vi "VNA_Interferometer.vi"() -> ()   [LabVIEW 2015]
doc: "Measure VNA FMR with interferometer circuit."
uses:
  <vilib>/Utility/file.llb/Read Delimited Spreadsheet (DBL).vi
  <vilib>/Utility/file.llb/Write Delimited Spreadsheet (DBL).vi
  <vilib>/Utility/file.llb/Write Delimited Spreadsheet (string).vi
panel:
  in  "Find fitting freq":bool
  in  "Fitting Freq":dbl=0.04650776797841169
  in  "Stopping":bool
  out "Field values":dbl[](array[numeric])
  out "Im values":dbl[](array[numeric])
  out "Re values":dbl[](array[numeric])
  in  "Polynomial Coefficients":dbl[](array[numeric])
  out "Max Field":dbl
  out "Time Remaining (min)":dbl
  out "Elapsed Time (min)":dbl caption="Elapsed Time (s)"
  in  "Trigger Delay (ms)":dbl=50.0
  in  "Burst Count":dbl=205.0
  in  "Modulation Frequency (Hz)":dbl=47.0
  in  "Amplitide (V)":dbl=5.0
  in  "SG GPIB Address":i16=22
  out "Total Points":dbl
  out "Field Set (Oe)":dbl
  in  "Start":bool
  out "Ready":bool
  in  "Stop":bool
  out "Status":string
  out "Measurement #":dbl
  out "Field Read (Oe)":dbl
  out "Email Errors":string
  out "Im Measurements":cluster{dbl[], dbl[]}(graph)
  out "Re Measurements":cluster{dbl[], dbl[]}(graph)
  out "Im VNA Output":cluster{"X-values":dbl[], "Input data":dbl[]}[](graph)
  in  "VNA Points":dbl=1000.0
  in  "VNA Power (dBm)":string="-17"
  in  "VNA GPIB Address":refnum<visa-resource-name>="GPIB0::15::INSTR"
  in  "VNA Frequency (GHz)":dbl=10.0
  in  "IF Bandwidth (Hz)":dbl=1000.0
  out "Re VNA Output":cluster{"X-values":dbl[], "Input data":dbl[]}[](graph)
  in  "Email Address":string
  in  "Send Email?":bool
  in  "File Name Comment":string
  in  "Save Directory":path=path "C:/Users/probe_station/Desktop/VNA_Interferometer_Data"
  in  "Gaussmeter GPIB Address":string="12"
  in  "Calibrate PS":bool
  in  "Stabilization Time (s)":dbl=5.0
  in  "Field Step (Oe)":dbl=10.0
  in  "Field Sweep Stop (Oe)":dbl=2000.0
  in  "Field Sweep Start (Oe)":dbl=5000.0
  in  "PS GPIB Address":string="1"
  # "Output Indicators"
  # "Timers"
  # "Signal Generator Controls"
  # "Program controls and status"
  # "VNA Controls"
  # "Output Controls"
  # "Field and Power Supply Controls"
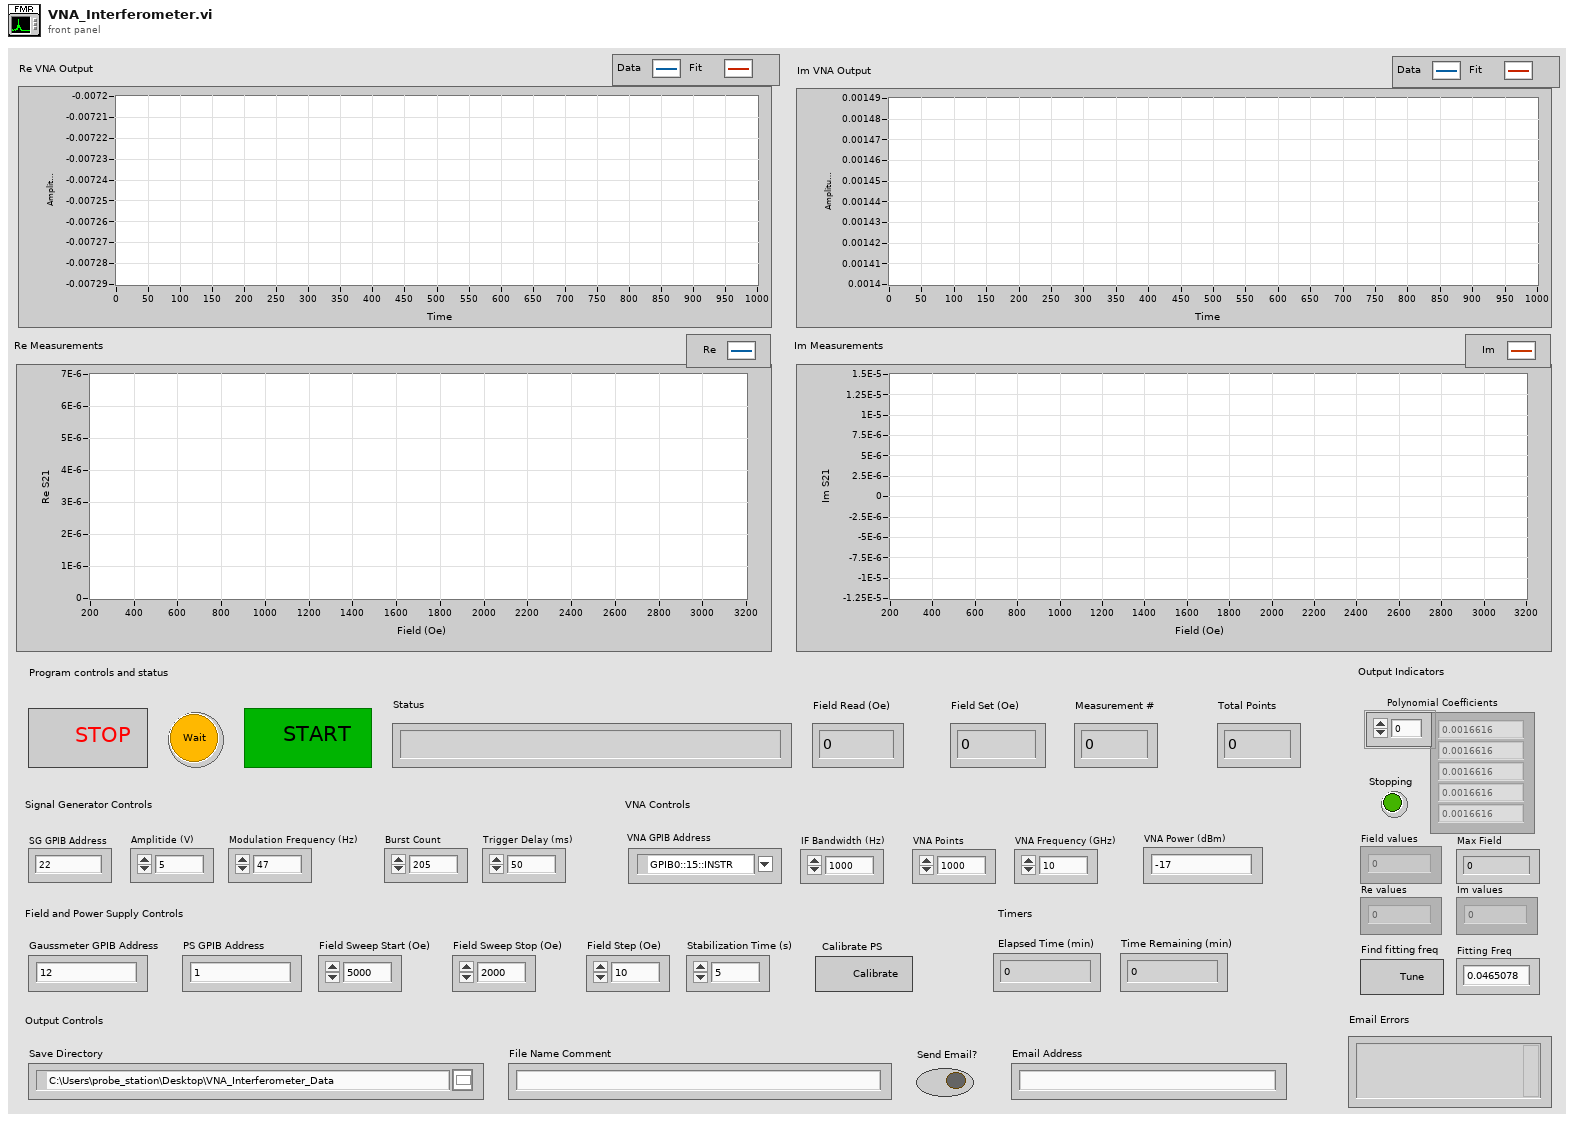
[diagram p1: front panel]
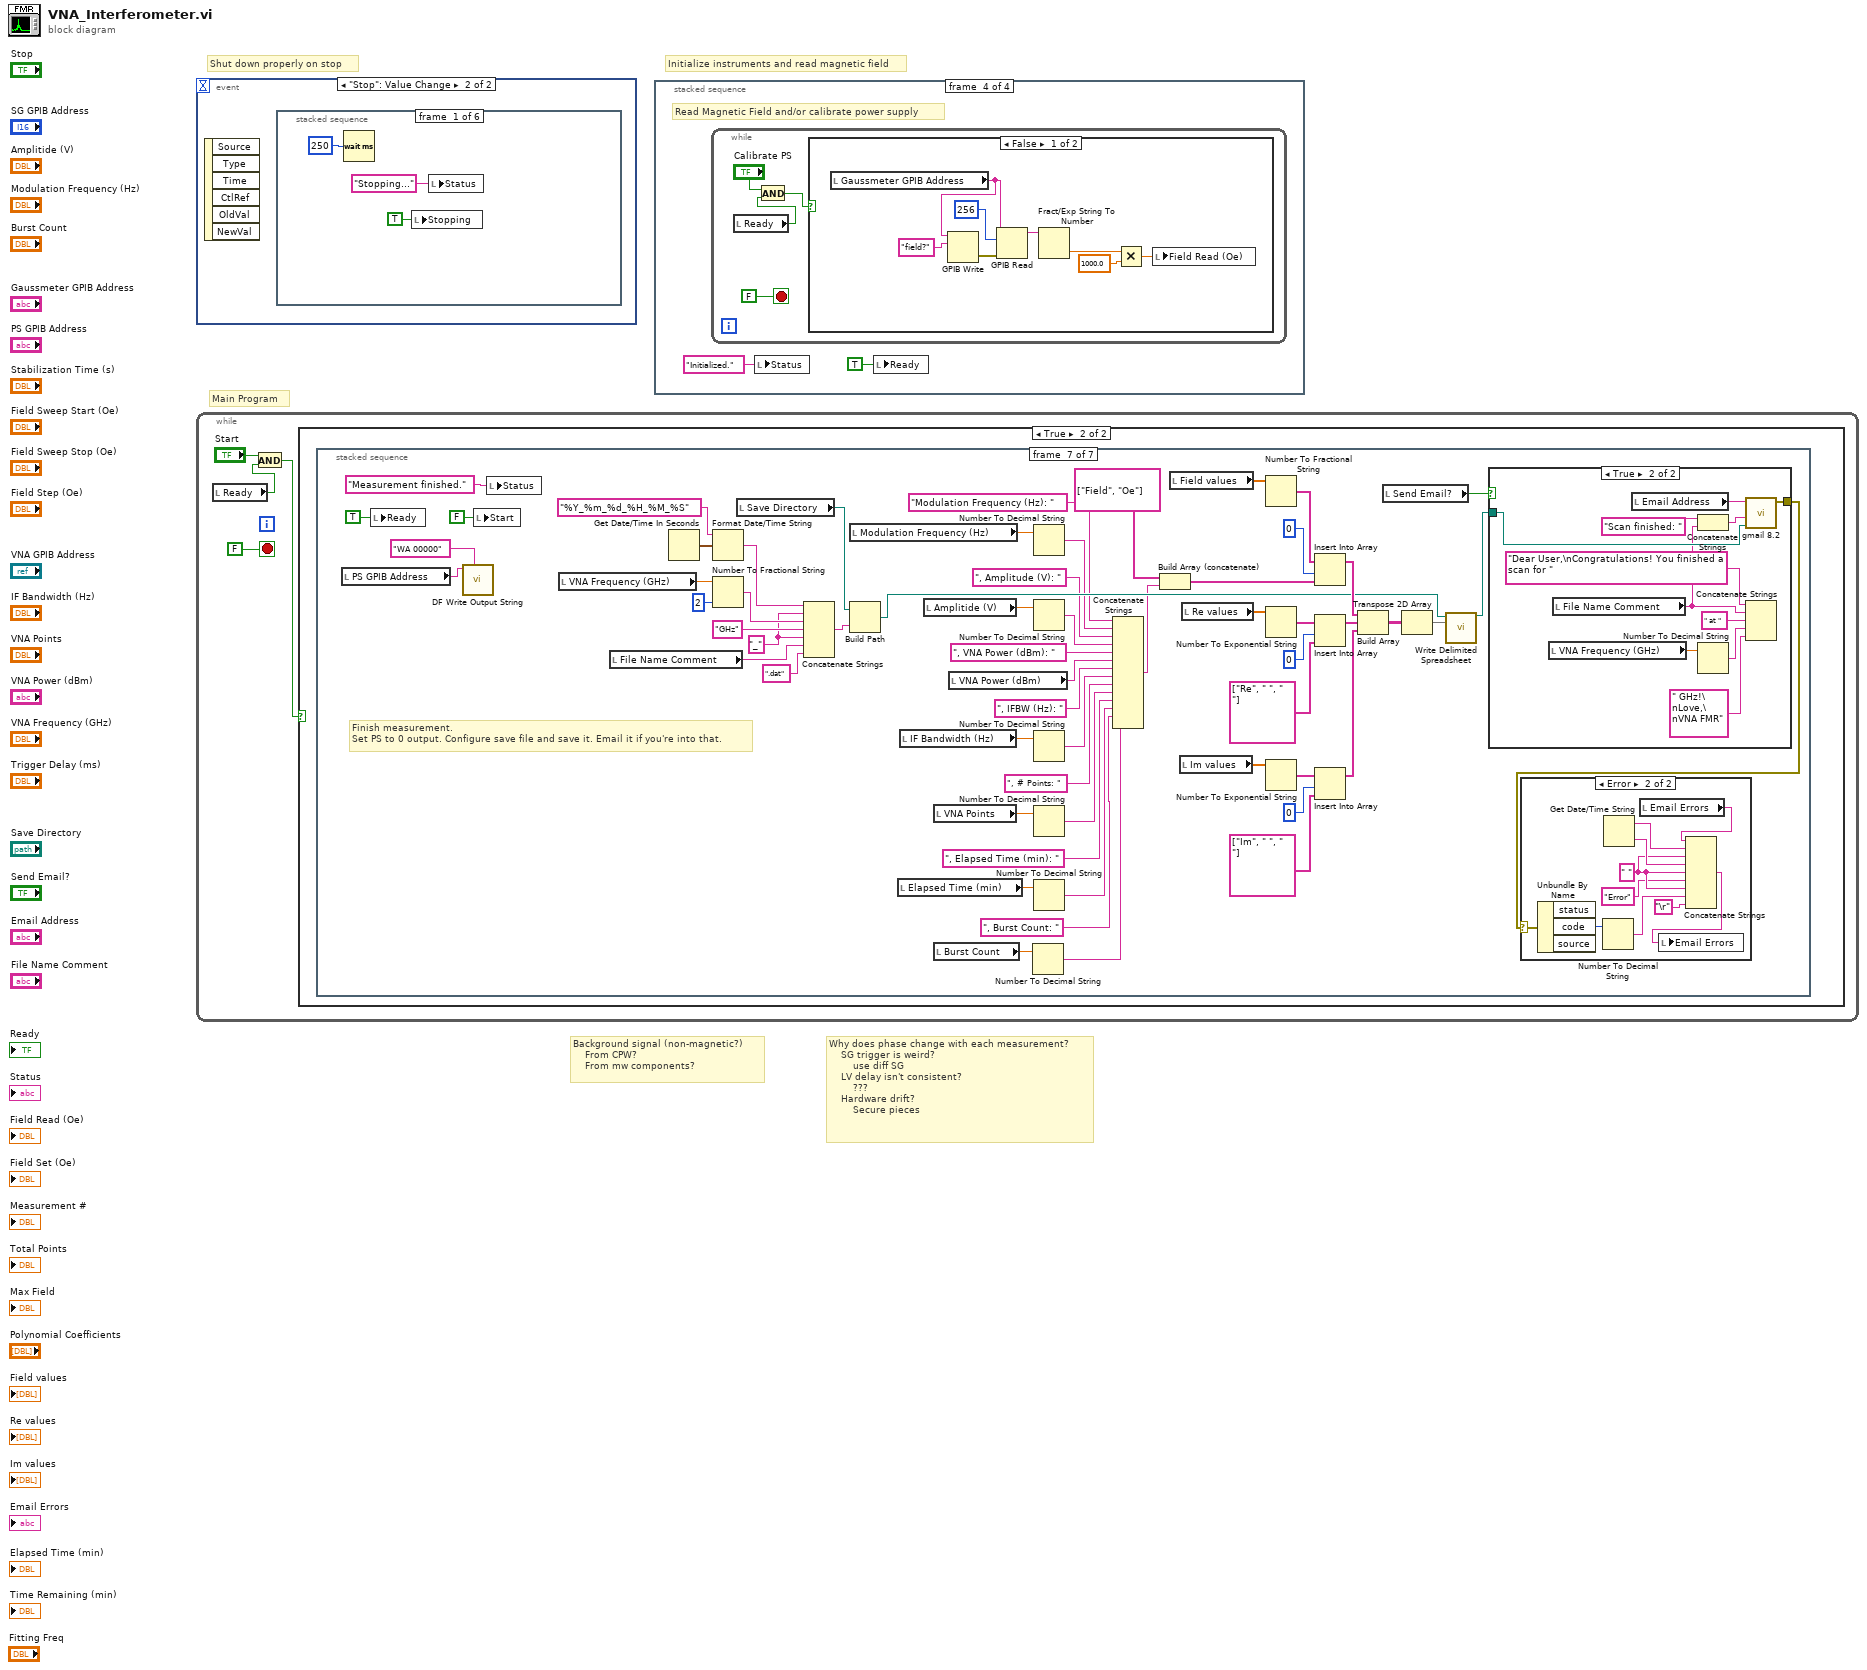
[diagram p0: block diagram]
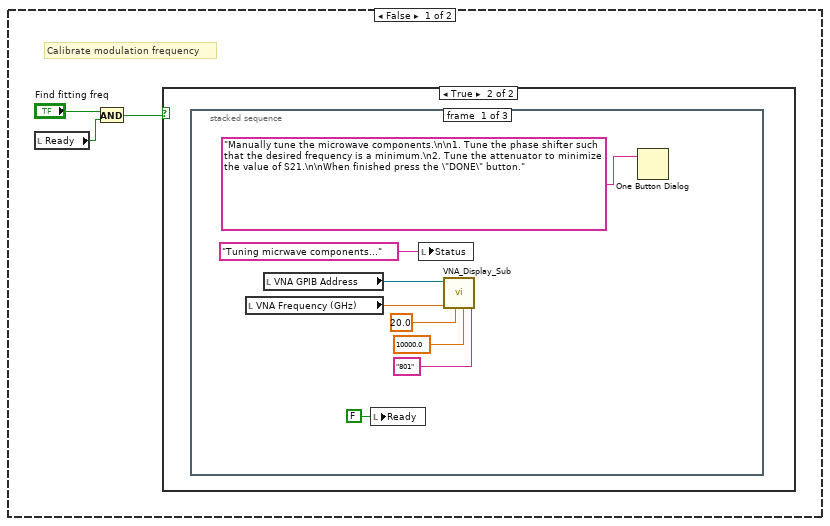
[diagram p2: hidden frame]
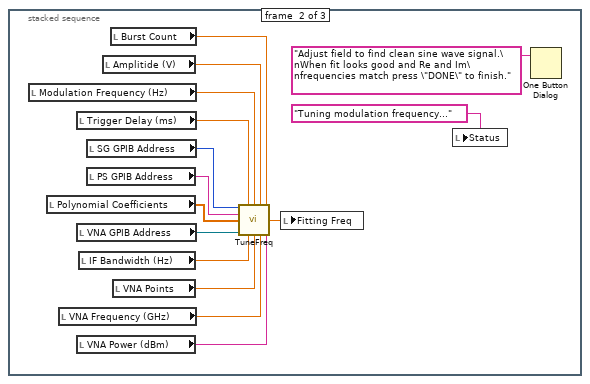
[diagram p4: hidden frame]
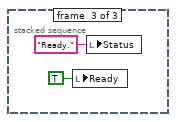
[diagram p5: hidden frame]
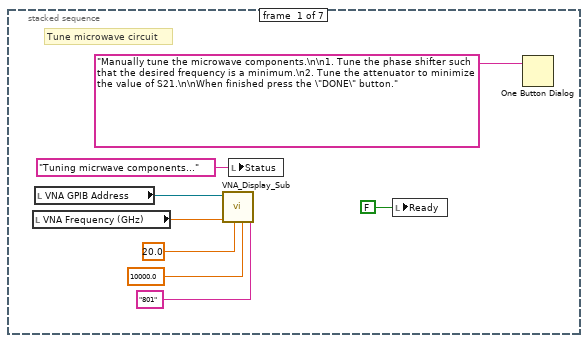
[diagram p6: hidden frame]
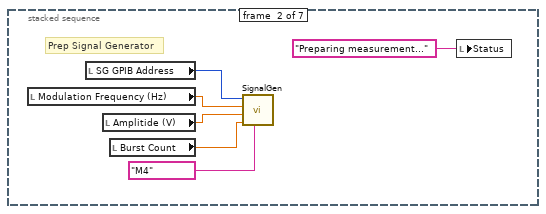
[diagram p7: hidden frame]
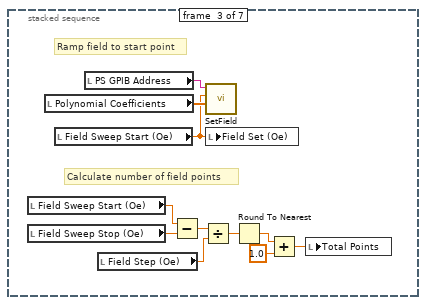
[diagram p8: hidden frame]
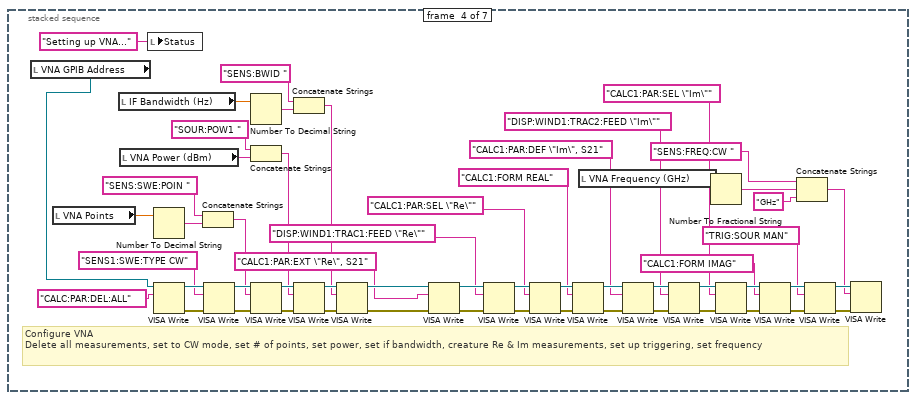
[diagram p9: hidden frame]
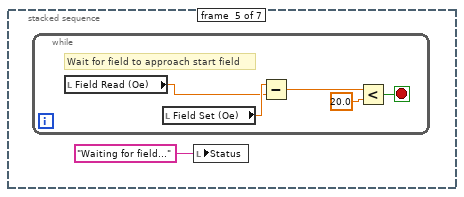
[diagram p10: hidden frame]
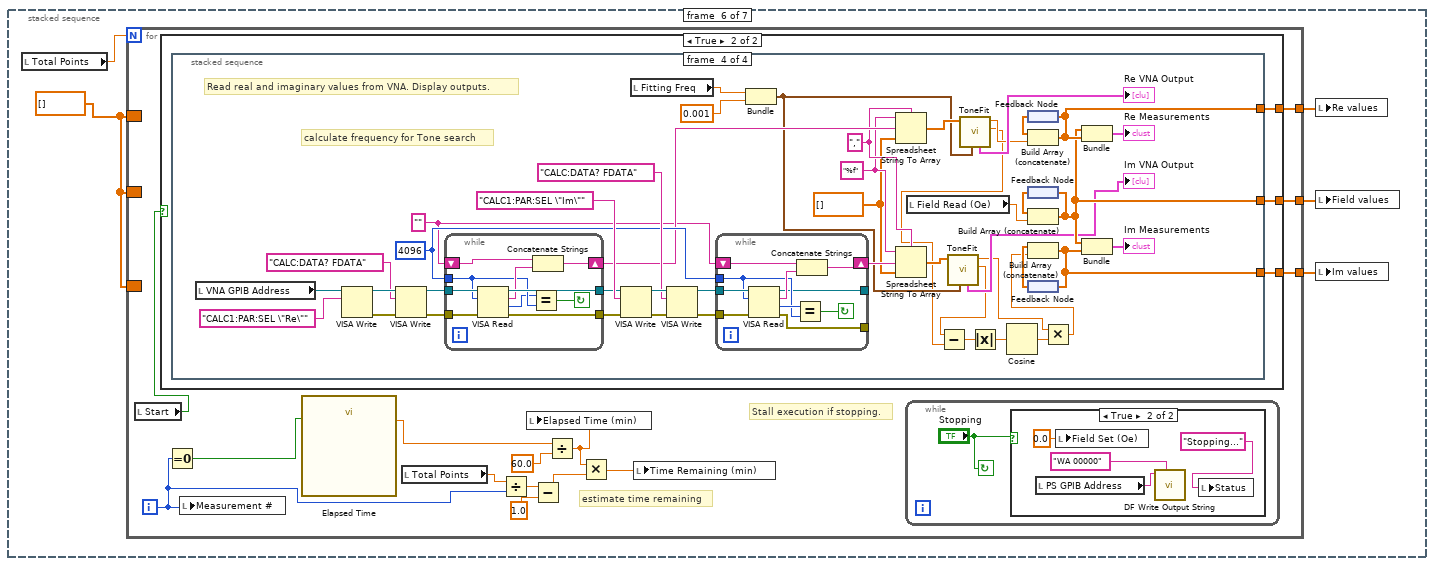
[diagram p11: hidden frame]
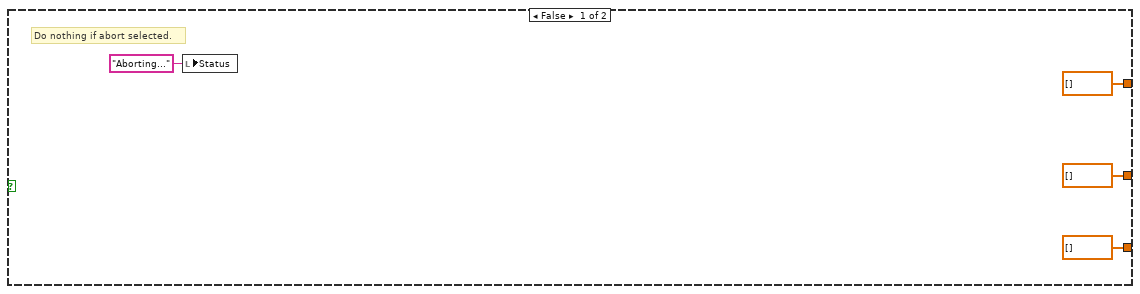
[diagram p12: hidden frame]
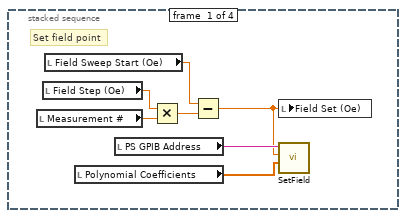
[diagram p13: hidden frame]
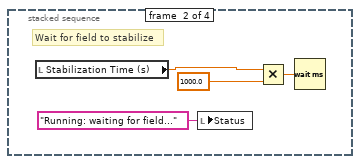
[diagram p14: hidden frame]
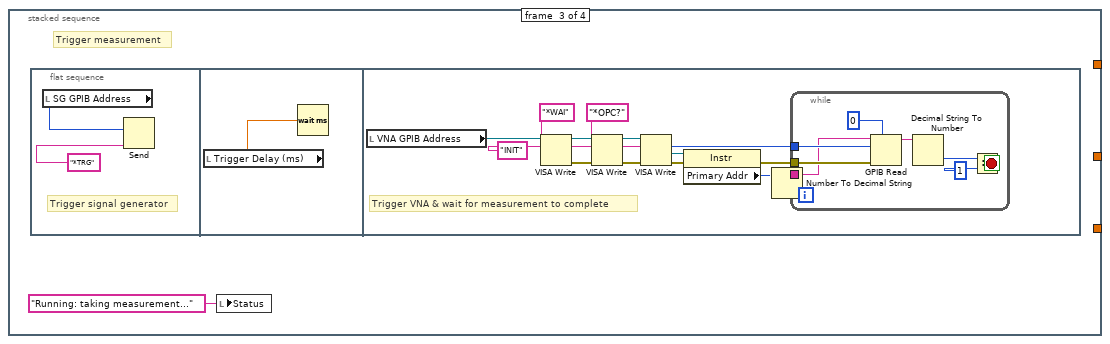
[diagram p15: hidden frame]
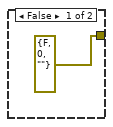
[diagram p18: hidden frame]
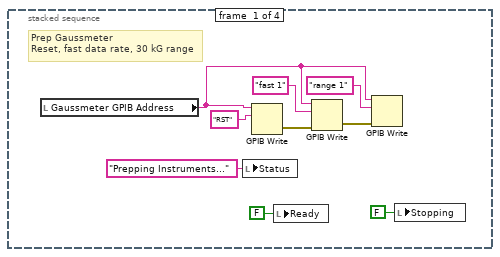
[diagram p19: hidden frame]
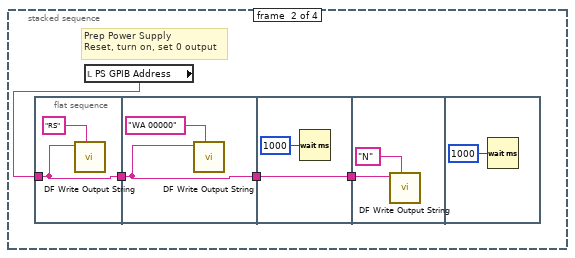
[diagram p20: hidden frame]
diagram:
  # "Background signal (non-magnetic?)\n    From CPW?\n    From mw components?"
  # "Why does phase change with each measurement?\n    SG trigger is weird?\n        use diff SG\n    LV delay isn't consistent?\n        ???\n    Hardware drift?\n        Secure pieces"
  # "Main Program"
  # "Initialize instruments and read magnetic field"
  # "Shut down properly on stop"
  n1 = event shown="[1] \"Stop\": Value Change" {
    selector: _ -> [_ _]
    dyn-events: _ -> [_ _]
    timeout: _ -> [_ _]
    event Timeout {
      n2 = event-data() -> ()  [unwired: 1 in, 3 out]
    }
    event "Stop": Value Change {
      n3 = event-data() -> ()  [unwired: 1 in, 6 out]
      n4 = stacked-sequence {
        frame #0 {
          n5 = Wait (ms)(milliseconds to wait=u32 250) -> ()  [unwired: 1 out]
          n6 = local write "Stopping"(TRUE ("Stopping")) -> ()
          n7 = local write "Status"("Stopping..." ("Status")) -> ()
        }
        frame #1 {
          # "Disable SG output"
          # "set power supply to 0 output"
          n8 = local read "PS GPIB Address"() -> (w7:string)
          n9 = local read "SG GPIB Address"() -> (w6:i16)
          n10 = call "DF Write Output String"("Write String"="WA 00000", "Communications Mode"=TRUE, "Communications On/Off"=TRUE, "GPIB Address"=w7) -> ()  [unwired: 5 in]
          n11 = Send(2:w6, 5:"D1" ("data string")) -> ()  [unwired: 3 in, 3 out]
          n12 = local write "Field Set (Oe)"(0.0 ("Field Set (Oe)")) -> ()
        }
        frame #2 {
          n13 = Wait (ms)(milliseconds to wait=u32 100) -> ()  [unwired: 1 out]
        }
        frame #3 {
          # "Wait for\nfield \nto reach\nzero"
          n14 = while {
            stop <- w12 stop-if-true
            n15 = local read "Field Read (Oe)"() -> (w14:dbl)
            n16 = Less?(x=w14, y=200.0) -> (x < y?=w12:bool)
          }
        }
        frame #4 {
          # "Turn off power supply"
          n17 = local read "PS GPIB Address"() -> (w15:string)
          n18 = local write "Status"("Stopped." ("Status")) -> ()
          n19 = call "DF Write Output String"("Write String"="F", "Communications Mode"=TRUE, "Communications On/Off"=TRUE, "GPIB Address"=w15) -> ()  [unwired: 5 in]
        }
        frame #5 {
          # "end program"
          n20 = Stop(stop? (T)=TRUE) -> ()
        }
      }
    }
  }
  n21 = while {
    stop <- FALSE stop-if-true
    n22 = local read "Ready"() -> (w23:bool)
    n23 = And(x="Start", y=w23) -> (x .and. y?=w22:bool)
    n24 = case shown="True" w22 {
      frame False {
        # "Calibrate modulation frequency"
        n25 = local read "Ready"() -> (w27:bool)
        n26 = And(x="Find fitting freq", y=w27) -> (x .and. y?=w25:bool)
        n27 = case shown="True" w25 {
          frame False {
          }
          frame True {
            n28 = stacked-sequence {
              frame #0 {
                n29 = local read "VNA Frequency (GHz)"() -> (w32:dbl)
                n30 = local read "VNA GPIB Address"() -> (w33:refnum<visa-resource-name>)
                n31 = local write "Ready"(FALSE ("Ready")) -> ()
                n32 = local write "Status"("Tuning micrwave components..." ("Status")) -> ()
                n33 = call "VNA_Display_Sub.vi"("Num points"="801", "IF Bandwidth"=10000.0, "Span Frequency (MHz)"=20.0, "Center Frequency (GHz)"=w32, "VNA Address"=w33) -> ()  [unwired: 7 in]
                n34 = One Button Dialog(message="Manually tune the microwave components.\n\n1. Tune the phase shifter such that the desired frequency is a minimum.\n2. Tune the attenuator to minimize the value of S21.\n\nWhen finished press the \"DONE\" button.") -> ()  [unwired: 1 in, 1 out]
              }
              frame #1 {
                n35 = local read "Modulation Frequency (Hz)"() -> (w41:dbl)
                n36 = local read "Polynomial Coefficients"() -> (w48:dbl[])
                n37 = local read "VNA Frequency (GHz)"() -> (w44:dbl)
                n38 = local read "Trigger Delay (ms)"() -> (w42:dbl)
                n39 = local read "VNA GPIB Address"() -> (w47:refnum<visa-resource-name>)
                n40 = local read "VNA Power (dBm)"() -> (w43:string)
                n41 = local read "IF Bandwidth (Hz)"() -> (w46:dbl)
                n42 = local read "SG GPIB Address"() -> (w50:i16)
                n43 = local read "PS GPIB Address"() -> (w49:string)
                n44 = local read "Amplitide (V)"() -> (w40:dbl)
                n45 = local read "Burst Count"() -> (w39:dbl)
                n46 = local read "VNA Points"() -> (w45:dbl)
                n47 = call "TuneFreq.vi"("SG GPIB Address"=w50, "Trigger Delay"=w42, "Mod Freq (Hz)"=w41, "Amplitude (V)"=w40, "Burst count"=w39, "PS GPIB Address"=w49, "Poly Coeffs"=w48, "VNA GPIB Address"=w47, "IF Bandwidth"=w46, "VNA Points"=w45, "VNA Frequency"=w44, "VNA Power (dBm)"=w43) -> ("Re Freq"=w38:dbl)  [unwired: 3 in]
                n48 = local write "Fitting Freq"(w38) -> ()
                n49 = local write "Status"("Tuning modulation frequency..." ("Status")) -> ()
                n50 = One Button Dialog(message="Adjust field to find clean sine wave signal.\nWhen fit looks good and Re and Im\nfrequencies match press \"DONE\" to finish.") -> ()  [unwired: 1 in, 1 out]
              }
              frame #2 {
                n51 = local write "Ready"(TRUE ("Ready")) -> ()
                n52 = local write "Status"("Ready." ("Status")) -> ()
              }
            }
          }
        }
      }
      frame True {
        n53 = stacked-sequence {
          frame #0 {
            # "Tune microwave circuit"
            n54 = local read "VNA Frequency (GHz)"() -> (w58:dbl)
            n55 = local read "VNA GPIB Address"() -> (w59:refnum<visa-resource-name>)
            n56 = call "VNA_Display_Sub.vi"("Num points"="801", "IF Bandwidth"=10000.0, "Span Frequency (MHz)"=20.0, "Center Frequency (GHz)"=w58, "VNA Address"=w59) -> ()  [unwired: 7 in]
            n57 = local write "Status"("Tuning micrwave components..." ("Status")) -> ()
            n58 = local write "Ready"(FALSE ("Ready")) -> ()
            n59 = One Button Dialog(message="Manually tune the microwave components.\n\n1. Tune the phase shifter such that the desired frequency is a minimum.\n2. Tune the attenuator to minimize the value of S21.\n\nWhen finished press the \"DONE\" button.") -> ()  [unwired: 1 in, 1 out]
          }
          frame #1 {
            # "Prep Signal Generator"
            n60 = local read "Modulation Frequency (Hz)"() -> (w65:dbl)
            n61 = local read "SG GPIB Address"() -> (w66:i16)
            n62 = local read "Amplitide (V)"() -> (w64:dbl)
            n63 = local read "Burst Count"() -> (w61:dbl)
            n64 = call "SignalGen.vi"("Trigger Mode (Cont)"="M4" ("Trigger Mode"), "Burst Count"=w61, "Amplitide (V)"=w64, "Modulation Frequency (Hz)"=w65, "SG GPIB Address"=w66) -> ()  [unwired: 7 in]
            n65 = local write "Status"("Preparing measurement..." ("Status")) -> ()
          }
          frame #2 {
            # "Calculate number of field points"
            # "Ramp field to start point"
            n66 = local read "Field Sweep Start (Oe)"() -> (w72:dbl)
            n67 = local read "Field Sweep Stop (Oe)"() -> (w71:dbl)
            n68 = local read "Polynomial Coefficients"() -> (w76:dbl[])
            n69 = local read "Field Sweep Start (Oe)"() -> (w75:dbl)
            n70 = local read "PS GPIB Address"() -> (w77:string)
            n71 = local read "Field Step (Oe)"() -> (w73:dbl)
            n72 = Subtract(x=w72, y=w71) -> (x-y=w74:dbl)
            n73 = Divide(x=w74, y=w73) -> (x/y=w70:dbl)
            n74 = call "SetField.vi"("Poly Coeffs"=w76, "Field Setpoint"=w75, "PS GPIB Address"=w77) -> ()  [unwired: 9 in]
            n75 = local write "Field Set (Oe)"(w75) -> ()
            n76 = Round To Nearest(number=w70) -> (nearest integer value=w69:dbl)
            n77 = Add(x=w69, y=1.0) -> (x+y=w67:dbl)
            n78 = local write "Total Points"(w67) -> ()
          }
          frame #3 {
            # "Configure VNA\nDelete all measurements, set to CW mode, set # of points, set power, set if bandwidth, creature Re & Im measurements, set up triggering, set frequency"
            n79 = local read "VNA GPIB Address"() -> (w86:refnum<visa-resource-name>)
            n80 = local read "VNA Points"() -> (w128:dbl)
            n81 = local read "IF Bandwidth (Hz)"() -> (w117:dbl)
            n82 = local read "VNA Power (dBm)"() -> (w122:string)
            n83 = local write "Status"("Setting up VNA..." ("Status")) -> ()
            n84 = Number To Decimal String(number=w128) -> (decimal integer string=w127:string)  [unwired: 1 in]
            n85 = VISA Write(VISA resource name=w86, write buffer="CALC:PAR:DEL:ALL" ("Characters to Write")) -> (VISA resource name out=w133:refnum<visa-resource-name>, error out=w87:errorcluster)  [unwired: 1 in, 1 out]
            n86 = Concatenate Strings("SENS:SWE:POIN " ("Characters to Write"), w127) -> (w126:string)
            n87 = VISA Write(VISA resource name=w133, write buffer="SENS1:SWE:TYPE CW" ("Characters to Write"), error in (no error)=w87) -> (VISA resource name out=w130:refnum<visa-resource-name>, error out=w131:errorcluster)  [unwired: 1 out]
            n88 = Number To Decimal String(number=w117) -> (decimal integer string=w116:string)  [unwired: 1 in]
            n89 = Concatenate Strings("SOUR:POW1 " ("Characters to Write"), w122) -> (w121:string)
            n90 = VISA Write(VISA resource name=w130, write buffer=w126, error in (no error)=w131) -> (VISA resource name out=w124:refnum<visa-resource-name>, error out=w125:errorcluster)  [unwired: 1 out]
            n91 = Concatenate Strings("SENS:BWID " ("Characters to Write"), w116) -> (w115:string)
            n92 = VISA Write(VISA resource name=w124, write buffer=w121, error in (no error)=w125) -> (VISA resource name out=w119:refnum<visa-resource-name>, error out=w120:errorcluster)  [unwired: 1 out]
            n93 = VISA Write(VISA resource name=w119, write buffer=w115, error in (no error)=w120) -> (VISA resource name out=w113:refnum<visa-resource-name>, error out=w114:errorcluster)  [unwired: 1 out]
            n94 = VISA Write(VISA resource name=w113, write buffer="CALC1:PAR:EXT \"Re\", S21" ("Characters to Write"), error in (no error)=w114) -> (VISA resource name out=w110:refnum<visa-resource-name>, error out=w111:errorcluster)  [unwired: 1 out]
            n95 = VISA Write(VISA resource name=w110, write buffer="DISP:WIND1:TRAC1:FEED \"Re\"" ("Characters to Write"), error in (no error)=w111) -> (VISA resource name out=w107:refnum<visa-resource-name>, error out=w108:errorcluster)  [unwired: 1 out]
            n96 = VISA Write(VISA resource name=w107, write buffer="CALC1:PAR:SEL \"Re\"" ("Characters to Write"), error in (no error)=w108) -> (VISA resource name out=w104:refnum<visa-resource-name>, error out=w105:errorcluster)  [unwired: 1 out]
            n97 = VISA Write(VISA resource name=w104, write buffer="CALC1:FORM REAL" ("Characters to Write"), error in (no error)=w105) -> (VISA resource name out=w101:refnum<visa-resource-name>, error out=w102:errorcluster)  [unwired: 1 out]
            n98 = local read "VNA Frequency (GHz)"() -> (w80:dbl)
            n99 = VISA Write(VISA resource name=w101, write buffer="CALC1:PAR:DEF \"Im\", S21" ("Characters to Write"), error in (no error)=w102) -> (VISA resource name out=w99:refnum<visa-resource-name>, error out=w98:errorcluster)  [unwired: 1 out]
            n100 = VISA Write(VISA resource name=w99, write buffer="DISP:WIND1:TRAC2:FEED \"Im\"" ("Characters to Write"), error in (no error)=w98) -> (VISA resource name out=w95:refnum<visa-resource-name>, error out=w96:errorcluster)  [unwired: 1 out]
            n101 = Number To Fractional String(number=w80) -> (F-format string=w81:string)  [unwired: 3 in]
            n102 = VISA Write(VISA resource name=w95, write buffer="CALC1:PAR:SEL \"Im\"" ("Characters to Write"), error in (no error)=w96) -> (VISA resource name out=w92:refnum<visa-resource-name>, error out=w93:errorcluster)  [unwired: 1 out]
            n103 = VISA Write(VISA resource name=w92, write buffer="CALC1:FORM IMAG" ("Characters to Write"), error in (no error)=w93) -> (VISA resource name out=w89:refnum<visa-resource-name>, error out=w90:errorcluster)  [unwired: 1 out]
            n104 = Concatenate Strings("SENS:FREQ:CW " ("Characters to Write"), w81, "GHz" ("string")) -> (w78:string)
            n105 = VISA Write(VISA resource name=w89, write buffer="TRIG:SOUR MAN", error in (no error)=w90) -> (VISA resource name out=w83:refnum<visa-resource-name>, error out=w84:errorcluster)  [unwired: 1 out]
            n106 = VISA Write(VISA resource name=w83, write buffer=w78, error in (no error)=w84) -> ()  [unwired: 3 out]
          }
          frame #4 {
            n107 = while {
              stop <- w139 stop-if-true
              # "Wait for field to approach start field"
              n108 = local read "Field Read (Oe)"() -> (w136:dbl)
              n109 = local read "Field Set (Oe)"() -> (w137:dbl)
              n110 = Subtract(x=w137, y=w136) -> (x-y=w138:dbl)
              n111 = Less?(x=w138, y=20.0) -> (x < y?=w139:bool)
            }
            n112 = local write "Status"("Waiting for field..." ("Status")) -> ()
          }
          frame #5 {
            w144 = dbl[] []
            n113 = local read "Total Points"() -> (w145:dbl)
            n114 = for {
              N: w145 -> [_]
              border: w144 -> [_]
              border: w144 -> [_]
              border: w144 -> [_]
              tunnel: [w159] -> w143
              tunnel: [w158] -> w142
              tunnel: [w157] -> w141
              i -> [w154]
              # "estimate time remaining"
              # "Stall execution if stopping."
              n115 = local read "Start"() -> (w156:bool)
              n116 = case shown="True" w156 {
                tunnel: [dbl[] [] w166] -> w159
                tunnel: [dbl[] [] w165] -> w158
                tunnel: [dbl[] [] w164] -> w157
                frame False {
                  # "Do nothing if abort selected."
                  n117 = local write "Status"("Aborting..." ("Status")) -> ()
                }
                frame True {
                  n118 = stacked-sequence {
                    tunnel: [_ _ _ w222] -> w166
                    tunnel: [_ _ _ w221] -> w165
                    tunnel: [_ _ _ w220] -> w164
                    frame #0 {
                      # "Set field point"
                      n119 = local read "Measurement #"() -> (w169:dbl)
                      n120 = local read "Field Step (Oe)"() -> (w168:dbl)
                      n121 = local read "Field Sweep Start (Oe)"() -> (w171:dbl)
                      n122 = local read "Polynomial Coefficients"() -> (w172:dbl[])
                      n123 = local read "PS GPIB Address"() -> (w173:string)
                      n124 = Multiply(x=w168, y=w169) -> (x*y=w170:dbl)
                      n125 = Subtract(x=w171, y=w170) -> (x-y=w167:dbl)
                      n126 = local write "Field Set (Oe)"(w167) -> ()
                      n127 = call "SetField.vi"("Poly Coeffs"=w172, "Field Setpoint"=w167, "PS GPIB Address"=w173) -> ()  [unwired: 9 in]
                    }
                    frame #1 {
                      # "Wait for field to stabilize"
                      n128 = local read "Stabilization Time (s)"() -> (w176:dbl)
                      n129 = local write "Status"("Running: waiting for field..." ("Status")) -> ()
                      n130 = Multiply(x=w176, y=1000.0) -> (x*y=w175:dbl)
                      n131 = Wait (ms)(milliseconds to wait=w175) -> ()  [unwired: 1 out]
                    }
                    frame #2 {
                      # "Trigger measurement"
                      n132 = flat-sequence {
                        frame #0 {
                          # "Trigger signal generator"
                          n133 = local read "SG GPIB Address"() -> (w180:i16)
                          n134 = Send(2:w180, 5:"*TRG") -> ()  [unwired: 3 in, 3 out]
                        }
                        frame #1 {
                          n135 = local read "Trigger Delay (ms)"() -> (w181:dbl)
                          n136 = Wait (ms)(milliseconds to wait=w181) -> ()  [unwired: 1 out]
                        }
                        frame #2 {
                          # "Trigger VNA & wait for measurement to complete"
                          n137 = local read "VNA GPIB Address"() -> (w194:refnum<visa-resource-name>)
                          n138 = VISA Write(VISA resource name=w194, write buffer="INIT") -> (VISA resource name out=w192:refnum<visa-resource-name>, error out=w191:errorcluster)  [unwired: 1 in, 1 out]
                          n139 = VISA Write(VISA resource name=w192, write buffer="*WAI", error in (no error)=w191) -> (VISA resource name out=w182:refnum<visa-resource-name>, error out=w189:errorcluster)  [unwired: 1 out]
                          n140 = VISA Write(VISA resource name=w182, write buffer="*OPC?", error in (no error)=w189) -> (VISA resource name out=w186:refnum<visa-resource-name>, return count=w188:u32, error out=w185:errorcluster)
                          n141 = property class="Instr"(reference=w186, error in=w185) -> (error out=w184:errorcluster, "Primary Addr"=w183:u16)  [unwired: 1 out]
                          n142 = Number To Decimal String(number=w183) -> (decimal integer string=w187:string)  [unwired: 1 in]
                          n143 = while {
                            tunnel: w184 -> [w199]
                            tunnel: w188 -> [w198]
                            tunnel: w187 -> [w196]
                            stop <- w201 stop-if-true
                            n144 = GPIB Read(0:w196, 1:w198, 3:w199, 4:0 ("timeout ms (488.2 global)")) -> (5:w200:string)  [unwired: 1 in, 2 out]
                            n145 = Decimal String To Number(string=w200) -> (number=w203:i32)  [unwired: 2 in, 1 out]
                            n146 = Equal?(x=w203, y=1) -> (x = y?=w201:bool)
                          }
                        }
                      }
                      n147 = local write "Status"("Running: taking measurement..." ("Status")) -> ()
                    }
                    frame #3 {
                      w223 = ""
                      w231 = dbl[] [] ("X")
                      w232 = "%f" ("format string")
                      w233 = "," ("delimiter (Tab)")
                      w237 = u32 4096
                      # "calculate frequency for Tone search"
                      # "Read real and imaginary values from VNA. Display outputs."
                      n148 = local read "VNA GPIB Address"() -> (w236:refnum<visa-resource-name>)
                      n149 = VISA Write(VISA resource name=w236, write buffer="CALC1:PAR:SEL \"Re\"" ("Characters to Write")) -> (VISA resource name out=w247:refnum<visa-resource-name>, error out=w248:errorcluster)  [unwired: 1 in, 1 out]
                      n150 = VISA Write(VISA resource name=w247, write buffer="CALC:DATA? FDATA", error in (no error)=w248) -> (VISA resource name out=w245:refnum<visa-resource-name>, error out=w244:errorcluster)  [unwired: 1 out]
                      n151 = while {
                        tunnel: w237 -> [w261]
                        tunnel: w245 -> [w269]
                        tunnel: [w266] -> w224
                        tunnel: w244 -> [w268]
                        tunnel: [w267] -> w225
                        shift-right: [w262] -> w235
                        shift-left: w223 -> [w263]
                        stop <- w265 continue-if-true
                        n152 = VISA Read(VISA resource name=w269, byte count=w261, error in (no error)=w268) -> (VISA resource name out=w266:refnum<visa-resource-name>, read buffer=w264:string, return count=w260:u32, error out=w267:errorcluster)
                        n153 = Equal?(x=w260, y=w261) -> (x = y?=w265:bool)
                        n154 = Concatenate Strings(w263, w264) -> (w262:string)
                      }
                      n155 = VISA Write(VISA resource name=w224, write buffer="CALC1:PAR:SEL \"Im\"" ("Characters to Write"), error in (no error)=w225) -> (VISA resource name out=w241:refnum<visa-resource-name>, error out=w242:errorcluster)  [unwired: 1 out]
                      n156 = local read "Fitting Freq"() -> (w206:dbl)
                      n157 = VISA Write(VISA resource name=w241, write buffer="CALC:DATA? FDATA", error in (no error)=w242) -> (VISA resource name out=w239:refnum<visa-resource-name>, error out=w238:errorcluster)  [unwired: 1 out]
                      n158 = while {
                        tunnel: w239 -> [w259]
                        tunnel: w238 -> [w258]
                        tunnel: w237 -> [w253]
                        shift-right: [w256] -> w234
                        shift-left: w223 -> [w255]
                        tunnel: [w251] -> _
                        tunnel: [w250] -> _
                        stop <- w252 continue-if-true
                        n159 = VISA Read(VISA resource name=w259, byte count=w253, error in (no error)=w258) -> (VISA resource name out=w251:refnum<visa-resource-name>, read buffer=w257:string, return count=w254:u32, error out=w250:errorcluster)
                        n160 = Equal?(x=w254, y=w253) -> (x = y?=w252:bool)
                        n161 = Concatenate Strings(w255, w257) -> (w256:string)
                      }
                      n162 = Bundle("Fitting Freq"=w206, "y"=0.001) -> (w208:cluster{"Fitting Freq":dbl, "y":dbl})  [unwired: 1 in]
                      n163 = Spreadsheet String To Array(delimiter (Tab)=w233, format string=w232, spreadsheet string=w235, array type (2D Dbl)=w231) -> (array=w214:dbl[])
                      n164 = Spreadsheet String To Array(delimiter (Tab)=w233, format string=w232, spreadsheet string=w234, array type (2D Dbl)=w231) -> (array=w211:dbl[])
                      n165 = local read "Field Read (Oe)"() -> (w229:dbl)
                      n166 = call "ToneFit.vi"("advanced search"=w208, "Input data"=w211) -> ("Phase"=w205:dbl, "Amplitude"=w207:dbl, "XY Graph"=→"Im VNA Output":cluster{"X-values":dbl[], "Input data":dbl[]}[])  [unwired: 6 in, 1 out]
                      n167 = call "ToneFit.vi"("advanced search"=w208, "Input data"=w214) -> ("Phase"=w204:dbl, "Amplitude"=w212:dbl, "XY Graph"=→"Re VNA Output":cluster{"X-values":dbl[], "Input data":dbl[]}[])  [unwired: 6 in, 1 out]
                      n168 = Subtract(x=w205, y=w204) -> (x-y=w218:dbl)
                      n169 = Absolute Value(x=w218) -> (abs(x)=w216:dbl)
                      n170 = Cosine(x=w216) -> (cos(x)=w217:dbl)
                      n171 = feedback #1() -> (w219:dbl[])
                      n172 = Build Array (concatenate)(w219, w212) -> (w222:dbl[])
                      n173 = feedback-in #1(w222) -> ()
                      n174 = feedback #2() -> (w228:dbl[])
                      n175 = Build Array (concatenate)(w228, w229) -> (w220:dbl[])
                      n176 = feedback-in #2(w220) -> ()
                      n177 = feedback #3() -> (w230:dbl[])
                      n178 = Multiply(x=w207, y=w217) -> (x*y=w209:dbl)
                      n179 = Build Array (concatenate)(w230, w209) -> (w221:dbl[])
                      n180 = feedback-in #3(w221) -> ()
                      n181 = Bundle(w220, w222) -> (→"Re Measurements":cluster{dbl[], dbl[]})  [unwired: 1 in]
                      n182 = Bundle(w220, w221) -> (→"Im Measurements":cluster{dbl[], dbl[]})  [unwired: 1 in]
                    }
                  }
                }
              }
              n183 = Equal To 0?(x=w154) -> (x = 0?=w155:bool)
              n184 = local write "Measurement #"(w154) -> ()
              n185 = call "Elapsed Time"("Reset"=w155) -> ("Elapsed Time (s)"=w149:dbl)  [unwired: 11 in, 7 out]
              n186 = local read "Total Points"() -> (w153:dbl)
              n187 = Divide(x=w153, y=w154) -> (x/y=w152:dbl)
              n188 = Subtract(x=w152, y=1.0) -> (x-y=w150:dbl)
              n189 = Divide(x=w149, y=60.0) -> (x/y=w146:dbl)
              n190 = local write "Elapsed Time (min)"(w146) -> ()
              n191 = Multiply(x=w146, y=w150) -> (x*y=w147:dbl)
              n192 = local write "Time Remaining (min)"(w147) -> ()
              n193 = while {
                stop <- "Stopping" continue-if-true
                n194 = case shown="True" "Stopping" {
                  frame False {
                  }
                  frame True {
                    n195 = local read "PS GPIB Address"() -> (w272:string)
                    n196 = local write "Field Set (Oe)"(0.0 ("Field Set (Oe)")) -> ()
                    n197 = call "DF Write Output String"("Write String"="WA 00000", "GPIB Address"=w272) -> ()  [unwired: 7 in]
                    n198 = local write "Status"("Stopping..." ("Status")) -> ()
                  }
                }
              }
            }
            n199 = local write "Re values"(w143) -> ()
            n200 = local write "Field values"(w141) -> ()
            n201 = local write "Im values"(w142) -> ()
          }
          frame #6 {
            w275 = "_" ("string")
            # "Finish measurement.\nSet PS to 0 output. Configure save file and save it. Email it if you're into that."
            n202 = local read "PS GPIB Address"() -> (w331:string)
            n203 = local write "Ready"(TRUE ("Ready")) -> ()
            n204 = call "DF Write Output String"("Write String"="WA 00000", "GPIB Address"=w331) -> ()  [unwired: 7 in]
            n205 = local write "Start"(FALSE ("Start")) -> ()
            n206 = local write "Status"("Measurement finished." ("Status")) -> ()
            n207 = local read "VNA Frequency (GHz)"() -> (w326:dbl)
            n208 = local read "File Name Comment"() -> (w277:string)
            n209 = Get Date/Time In Seconds() -> (seconds since 1Jan1904=w329:timestamp)
            n210 = Format Date/Time String(time format string (%c)="%Y_%m_%d_%H_%M_%S", seconds (now)=w329) -> (date/time string=w327:string)  [unwired: 1 in]
            n211 = Number To Fractional String(number=w326, precision (6)=i16 2) -> (F-format string=w325:string)  [unwired: 2 in]
            n212 = local read "Save Directory"() -> (w324:path)
            n213 = Concatenate Strings(w327, w275, w325, "GHz" ("string"), w275, w277, ".dat" ("string")) -> (w323:string)
            n214 = local read "Modulation Frequency (Hz)"() -> (w303:dbl)
            n215 = Build Path(base path=w324, name or relative path=w323) -> (appended path=w307:path)
            n216 = local read "Elapsed Time (min)"() -> (w283:dbl)
            n217 = local read "IF Bandwidth (Hz)"() -> (w295:dbl)
            n218 = local read "Amplitide (V)"() -> (w300:dbl)
            n219 = local read "VNA Points"() -> (w292:dbl)
            n220 = local read "Burst Count"() -> (w281:dbl)
            n221 = local read "VNA Power (dBm)"() -> (w297:string)
            n222 = Number To Decimal String(number=w281) -> (decimal integer string=w279:string)  [unwired: 1 in]
            n223 = Number To Decimal String(number=w303) -> (decimal integer string=w302:string)  [unwired: 1 in]
            n224 = Number To Decimal String(number=w300) -> (decimal integer string=w299:string)  [unwired: 1 in]
            n225 = Number To Decimal String(number=w295) -> (decimal integer string=w294:string)  [unwired: 1 in]
            n226 = Number To Decimal String(number=w292) -> (decimal integer string=w291:string)  [unwired: 1 in]
            n227 = Number To Decimal String(number=w283) -> (decimal integer string=w282:string)  [unwired: 1 in]
            n228 = Concatenate Strings("Modulation Frequency (Hz): " ("string"), w302, ", Amplitude (V): " ("string"), w299, ", VNA Power (dBm): " ("string"), w297, ", IFBW (Hz): " ("string"), w294, ", # Points: " ("string"), w291, ", Elapsed Time (min): " ("string"), w282, ", Burst Count: " ("string"), w279) -> (w290:string)
            n229 = Build Array (concatenate)(string[] ["Field", "Oe"] ("new element/subarray"), w290) -> (w289:string[])
            n230 = local read "Field values"() -> (w311:dbl[])
            n231 = local read "Im values"() -> (w322:dbl[])
            n232 = local read "Re values"() -> (w312:dbl[])
            n233 = Number To Fractional String(number=w311) -> (F-format string=w314:string[])  [unwired: 3 in]
            n234 = Number To Exponential String(number=w312) -> (E-format string=w317:string[])  [unwired: 3 in]
            n235 = Number To Exponential String(number=w322) -> (E-format string=w321:string[])  [unwired: 3 in]
            n236 = Insert Into Array(array=w314, index=0, new element=w289) -> (w310:string[])
            n237 = Insert Into Array(array=w317, index=0, new element=string[] ["Re", " ", " "] ("F-format string")) -> (w309:string[])
            n238 = Insert Into Array(array=w321, index=0, new element=string[] ["Im", " ", " "] ("F-format string")) -> (w318:string[])
            n239 = Build Array(w310, w309, w318) -> (w330:string[][])
            n240 = local read "Send Email?"() -> (w288:bool)
            n241 = Transpose 2D Array(2D array=w330) -> (transposed array=w308:string[][])
            n242 = call-poly <vilib>:"Write Delimited Spreadsheet.vi"("file path (dialog if empty)"=w307, "2D data"=w308) -> ("new file path (Not A Path if cancelled)"=w287:path)  [unwired: 12 in, 1 out]
            n243 = case shown="True" w288 {
              tunnel: w287 -> [_ w353]
              tunnel: [errorcluster {"status"=FALSE, "code"=0, "source"=""} ("error out") w346] -> w286
              frame False {
              }
              frame True {
                n244 = local read "VNA Frequency (GHz)"() -> (w349:dbl)
                n245 = local read "File Name Comment"() -> (w351:string)
                n246 = local read "Email Address"() -> (w356:string)
                n247 = Concatenate Strings("Scan finished: " ("string"), w351) -> (w354:string)
                n248 = Number To Decimal String(number=w349) -> (decimal integer string=w348:string)  [unwired: 1 in]
                n249 = call "gmail 8.2.vi"("Attachment - Optional"=w353, "Subject"=w354, "Recipient's Email Address Address"=w356) -> ("error out"=w346:errorcluster)  [unwired: 8 in]
                n250 = Concatenate Strings("Dear User,\nCongratulations! You finished a scan for " ("string"), w351, " at " ("string"), w348, " GHz!\nLove,\nVNA FMR" ("string")) -> ()  [unwired: 1 out]
              }
            }
            n251 = case shown="Error" w286 {
              selector: w286 -> [_ w344]
              frame No Error {
              }
              frame Error {
                w338 = " " ("string")
                n252 = Unbundle By Name(w344) -> ("code"=w341:i32)  [unwired: 2 out]
                n253 = Number To Decimal String(number=w341) -> (decimal integer string=w340:string)  [unwired: 1 in]
                n254 = Get Date/Time String() -> (date string=w343:string, time string=w342:string)  [unwired: 3 in]
                n255 = local read "Email Errors"() -> (w335:string)
                n256 = Concatenate Strings(w335, w343, w338, w342, w338, "Error" ("string"), w338, w340, "\r") -> (w336:string)
                n257 = local write "Email Errors"(w336) -> ()
              }
            }
          }
        }
      }
    }
  }
  n258 = stacked-sequence {
    frame #0 {
      # "Prep Gaussmeter\nReset, fast data rate, 30 kG range"
      n259 = local read "Gaussmeter GPIB Address"() -> (w365:string)
      n260 = local write "Status"("Prepping Instruments..." ("Status")) -> ()
      n261 = GPIB Write(0:w365, 1:"RST" ("data")) -> (6:w358:errorcluster)  [unwired: 3 in, 1 out]
      n262 = local write "Ready"(FALSE ("Ready")) -> ()
      n263 = GPIB Write(0:w365, 1:"fast 1" ("data"), 3:w358) -> (6:w362:errorcluster)  [unwired: 2 in, 1 out]
      n264 = GPIB Write(0:w365, 1:"range 1" ("data"), 3:w362) -> ()  [unwired: 2 in, 2 out]
      n265 = local write "Stopping"(FALSE ("Stopping")) -> ()
    }
    frame #1 {
      # "Prep Power Supply\nReset, turn on, set 0 output"
      n266 = flat-sequence {
        tunnel: w369 -> [w370]
        tunnel: [w370] -> w368
        tunnel: w368 -> [w372]
        tunnel: [w372] -> w367
        tunnel: w367 -> [w375]
        tunnel: [w375] -> w366
        tunnel: w366 -> [w376]
        frame #0 {
          n267 = call "DF Write Output String"("Write String"="RS", "GPIB Address"=w370) -> ()  [unwired: 7 in]
        }
        frame #1 {
          n268 = call "DF Write Output String"("Write String"="WA 00000", "GPIB Address"=w372) -> ()  [unwired: 7 in]
        }
        frame #2 {
          n269 = Wait (ms)(milliseconds to wait=u32 1000) -> ()  [unwired: 1 out]
        }
        frame #3 {
          n270 = call "DF Write Output String"("Write String"="N", "GPIB Address"=w376) -> ()  [unwired: 7 in]
        }
        frame #4 {
          n271 = Wait (ms)(milliseconds to wait=u32 1000) -> ()  [unwired: 1 out]
        }
      }
      n272 = local read "PS GPIB Address"() -> (w369:string)
    }
    frame #2 {
      # "Load PS calibration coefficients"
      n273 = call-poly <vilib>:"Read Delimited Spreadsheet.vi"("file path (dialog if empty)"=path "C:/VNA-FMR user/Desktop/Labview/VNA Modulation/PScal.dat", "format (%.3f)"="%g") -> ("all rows"=w381:dbl[][])  [unwired: 8 in, 5 out]
      n274 = Index Array(array=w381, index (row)=0 ("disabled index (col)")) -> (element=w380:dbl[])  [unwired: 1 in]
      n275 = local write "Polynomial Coefficients"(w380) -> ()
    }
    frame #3 {
      # "Read Magnetic Field and/or calibrate power supply"
      n276 = while {
        stop <- FALSE stop-if-true
        n277 = local read "Ready"() -> (w389:bool)
        n278 = And(x="Calibrate PS", y=w389) -> (x .and. y?=w388:bool)
        n279 = case shown="False" w388 {
          frame False {
            n280 = local read "Gaussmeter GPIB Address"() -> (w395:string)
            n281 = GPIB Write(0:w395, 1:"field?" ("data")) -> (6:w396:errorcluster)  [unwired: 3 in, 1 out]
            n282 = GPIB Read(0:w395, 1:256 ("byte count"), 3:w396) -> (5:w394:string)  [unwired: 2 in, 2 out]
            n283 = Fract/Exp String To Number(string=w394) -> (number=w391:dbl)  [unwired: 3 in, 1 out]
            n284 = Multiply(x=w391, y=1000.0) -> (x*y=w390:dbl)
            n285 = local write "Field Read (Oe)"(w390) -> ()
          }
          frame True {
            n286 = stacked-sequence {
              frame #0 {
                n287 = local read "Gaussmeter GPIB Address"() -> (w403:string)
                n288 = local read "PS GPIB Address"() -> (w404:string)
                n289 = call "CalPSv2.vi"("Gaussmeter GPIB Address"=w403, "PS GPIB Address"=w404) -> ("Max Field (Oe)"=w400:dbl, "Polynomial Coefficients"=w402:dbl[])  [unwired: 8 in]
                n290 = local write "Polynomial Coefficients"(w402) -> ()
                n291 = local write "Status"("Calibrating power supply..." ("Status")) -> ()
                n292 = local write "Max Field"(w400) -> ()
                n293 = One Button Dialog(message="Wait for PS to ramp then ensure fit is good.\nPress \"DONE\" button when finished.") -> ()  [unwired: 1 in, 1 out]
                n294 = local write "Ready"(FALSE ("Ready")) -> ()
              }
              frame #1 {
                # "write coeffs, set 0 output"
                n295 = local read "Polynomial Coefficients"() -> (w411:dbl[])
                n296 = call-poly <vilib>:"Write Delimited Spreadsheet.vi"("file path (dialog if empty)"=path "C:/VNA-FMR user/Desktop/Labview/VNA Modulation/PScal.dat", "format (%.3f)"="%g", "1D data"=w411) -> ()  [unwired: 11 in, 2 out]
                n297 = local write "Status"("Calibration finished." ("Status")) -> ()
                n298 = local read "PS GPIB Address"() -> (w407:string)
                n299 = local write "Ready"(TRUE ("Ready")) -> ()
                n300 = call "DF Write Output String"("Write String"="WA 00000", "GPIB Address"=w407) -> ()  [unwired: 7 in]
              }
            }
          }
        }
      }
      n301 = local write "Status"("Initialized." ("Status")) -> ()
      n302 = local write "Ready"(TRUE ("Ready")) -> ()
    }
  }
